vi "Main.vi"(11 "Module Admin":refnum<class "Delacor_lib_QMH_Cloneable Module Admin.lvclass">) -> ()   [LabVIEW 2020, in "DAQ AI.lvlib"]
doc: "This template is based off of the Queued Message Handler design pattern and the Queued Message Handler project template that ships with LabVIEW.\n\nThe main difference is that the queue is private to this module and communication between modules is performed via Broadcast and Request events.\n\nRequest events are wrapped in public API methods and are handled in the Event Handling Loop (EHL) of this VI. Any module can register for Broadcast events sent by this module. The EHL generates messages based on user interface actions.\n\nThe Message Handling Loop (MHL) processes messages generated by the EHL, or by other messages. The messages are string values, so new messages can be added easily to the Message Cases case structure in the MHL. Each message cluster can also provide an optional value for Message Data, which is a variant that can be converted to whatever message-specific data is required.\n_____\nBased on DQMH Dev Tools: Project Template 7.1.2.1547."
uses:
  DAQ AI.lvlib
  <vilib>/Delacor/Delacor QMH/Libraries/Cloneable Module Admin_class/Delacor_lib_QMH_Cloneable Module Admin.lvclass
  <vilib>/Delacor/Delacor QMH/Libraries/Message Queue_class/Delacor_lib_QMH_Message Queue.lvclass
  Module Data--cluster.ctl
  <vilib>/Utility/miscctls.llb/LVPointTypeDef.ctl
  <vilib>/Delacor/Delacor QMH/Libraries/Message Queue_class/Delacor_lib_QMH_Enqueue Message (Single).vi
  Stop Argument--cluster.ctl
  Get DAQ Analog Channel Argument--cluster.ctl
  <vilib>/DAQmx/read.llb/DAQmx Read (Analog DBL 1Chan 1Samp).vi
  Stop Acquisition Argument--cluster.ctl
  <vilib>/DAQmx/create/channels.llb/DAQmx Create Channel (AI-Voltage-Basic).vi
panel:
  out "task out":refnum<k21>
  out "DAQmx Physical Channel":tag
  out "error out":errorcluster
  out "Status":string
  in  "Simulate EHL Error":bool
  in  "Simulate MHL Error":bool
  # "Other processes communicate with this Module via its Public API (wrappers for its Request Events).\n\nThis Module communicates with other processes via its Broadcast Events.\nAny process that wants to receive these messages can register for this module's Broadcast events."
  # "This template is for the DQMH framework. See the block diagram for more information on how to use this template."
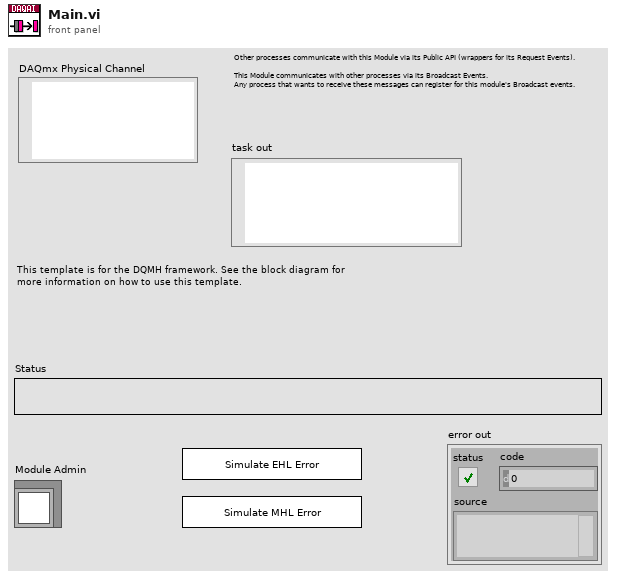
[diagram p1: front panel]
types:
  T1 = typedef "DAQ AI.lvlib/Request Events--cluster.ctl" = cluster{"Stop Module":refnum<user-event>, "Show Panel":refnum<user-event>, "Hide Panel":refnum<user-event>, "Show Diagram":refnum<user-event>, "Get Module Execution Status":refnum<user-event>, "Get DAQ Analog Channel":refnum<user-event>, "Get Acquisition Period":refnum<user-event>, "Stop Acquisition":refnum<user-event>}
  T2 = typedef "DAQ AI.lvlib/Module Data--cluster.ctl" = cluster{"Status":string, "DAQ Task":refnum<k21>}
  T3 = enum32{"invalid lock state", "Not Locked", "Locked (No Password)", "Password-protected"}
  T4 = typedef "DAQ AI.lvlib/Stop Argument--cluster.ctl" = cluster{"Module ID":i32, "Origin":string, "Exit via Stop Module Req?":bool, "Wait for Module to stop?":bool}
  T5 = typedef "DAQ AI.lvlib/Get DAQ Analog Channel Argument--cluster.ctl" = cluster{"Module ID":i32, "DAQmx Physical Channel":tag}
  T6 = typedef "DAQ AI.lvlib/Stop Acquisition Argument--cluster.ctl" = cluster{"Module ID":i32, "Dummy":bool}
  T7 = typedef "LVPointTypeDef.ctl" = cluster{"Horizontal":i16, "Vertical":i16}
  T8 = enum32{"Invalid", "Standard", "Closed", "Hidden", "Minimized", "Maximized"}
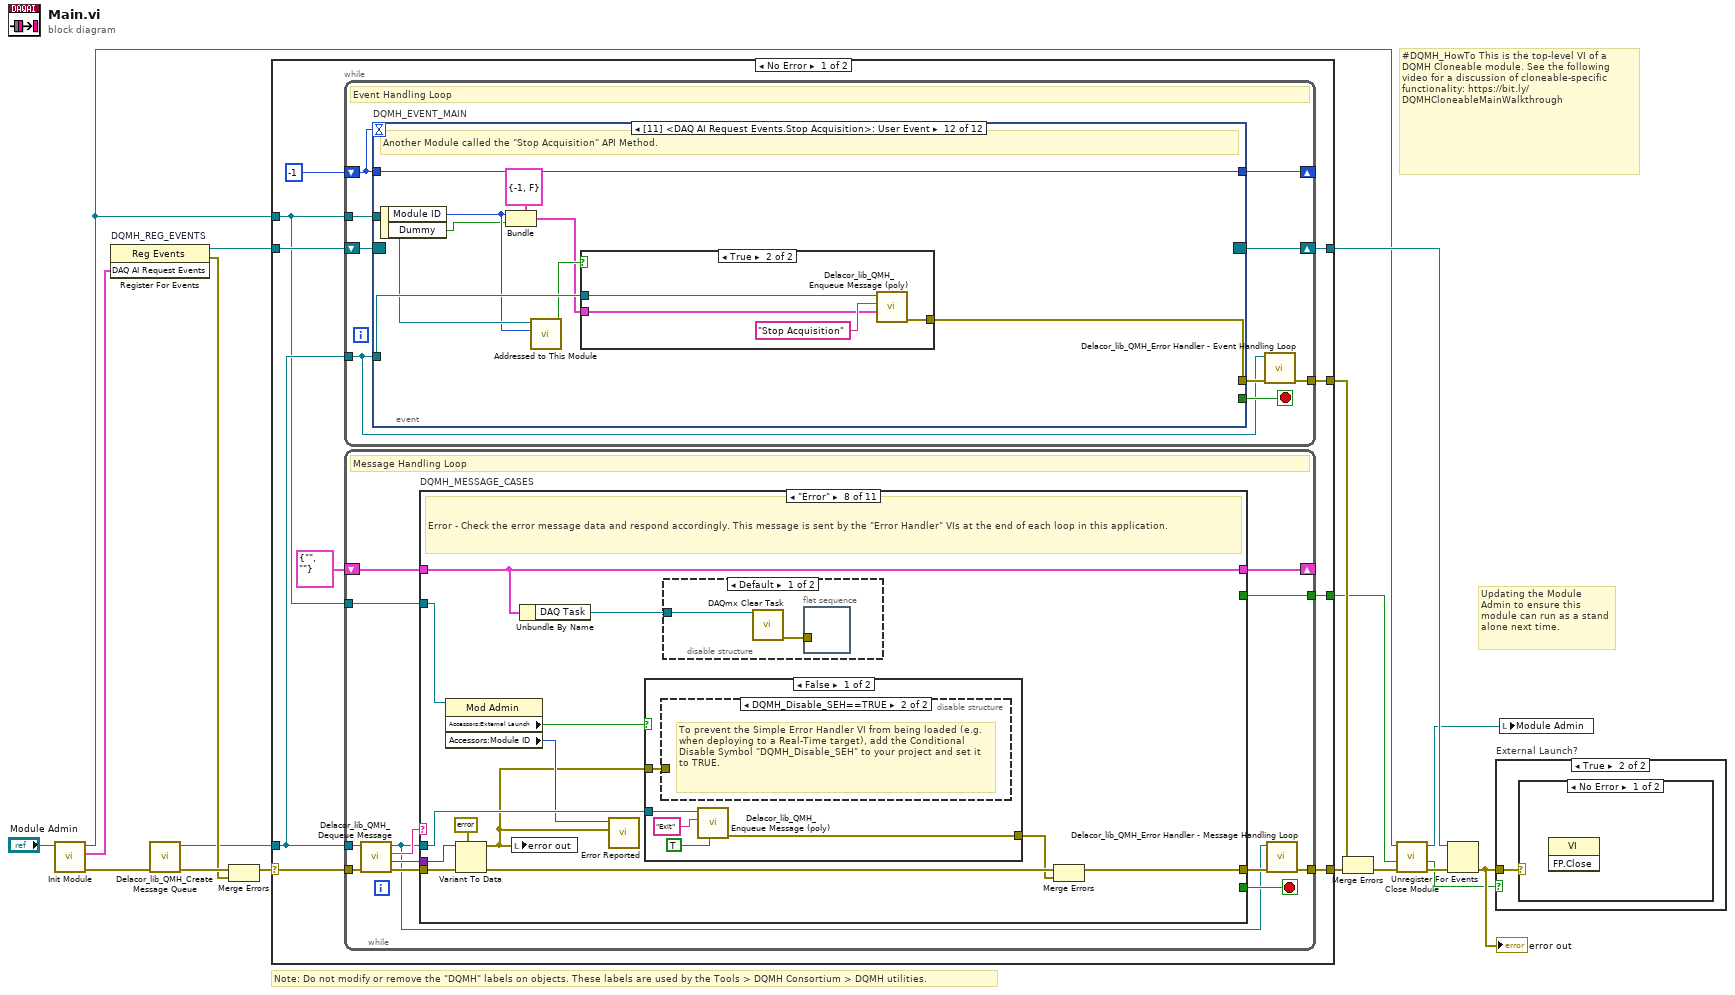
[diagram p0: block diagram]
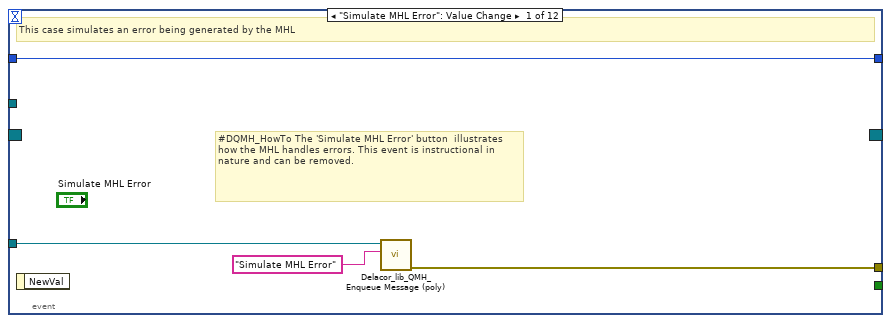
[diagram p2: hidden frame]
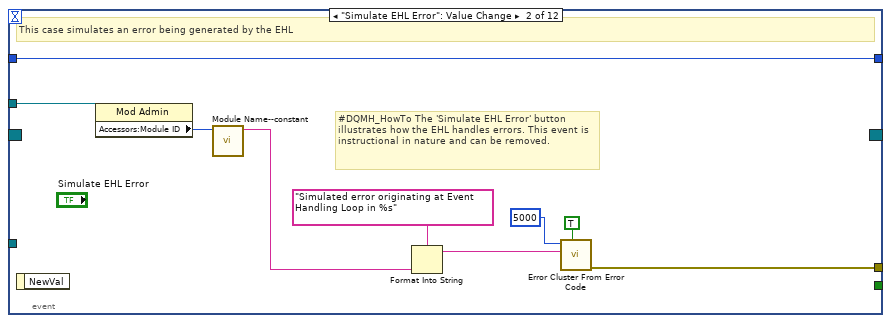
[diagram p3: hidden frame]
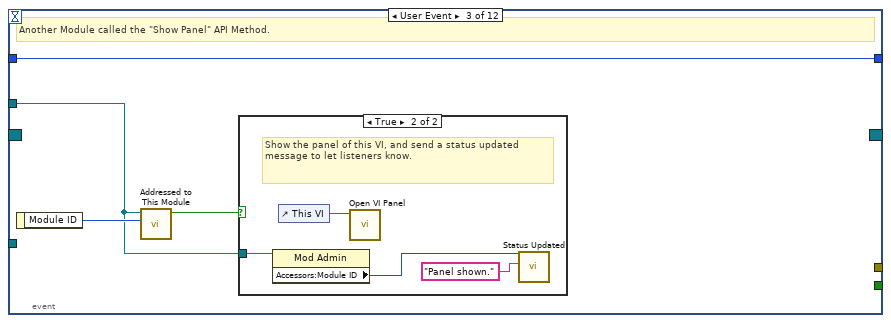
[diagram p4: hidden frame]
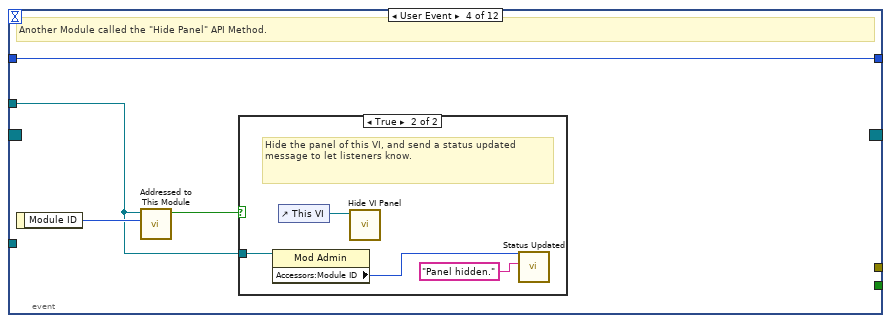
[diagram p6: hidden frame]
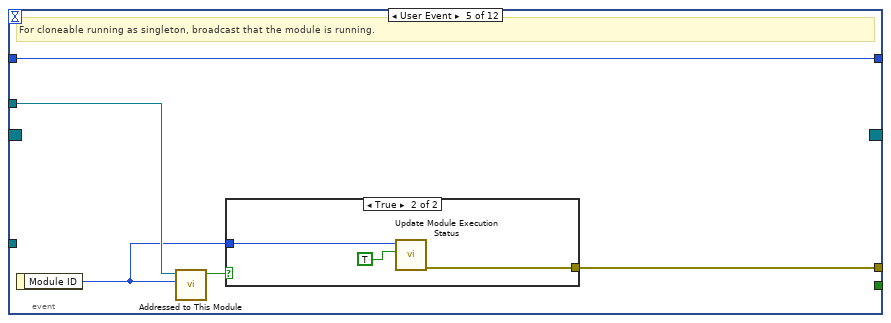
[diagram p8: hidden frame]
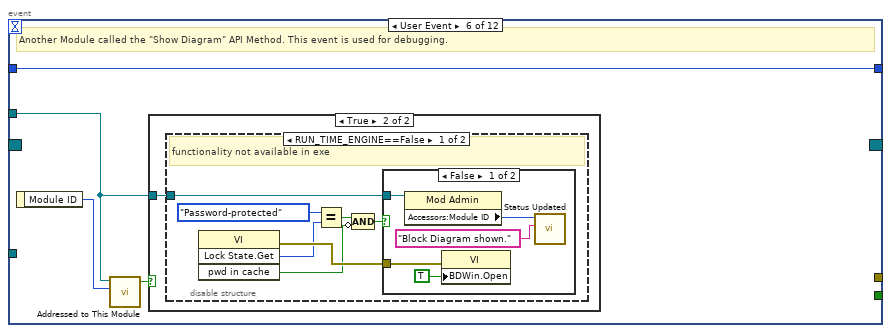
[diagram p10: hidden frame]
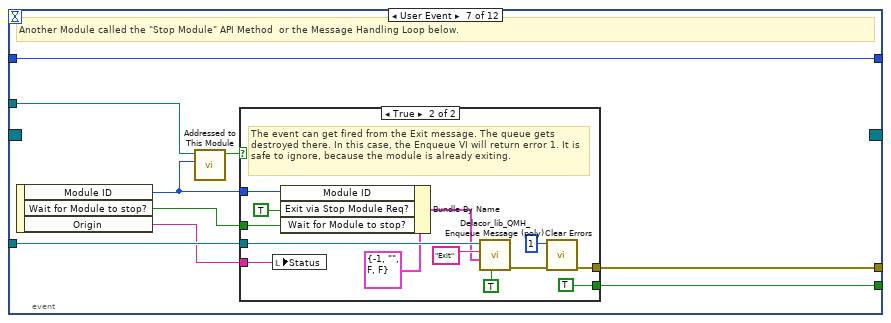
[diagram p14: hidden frame]
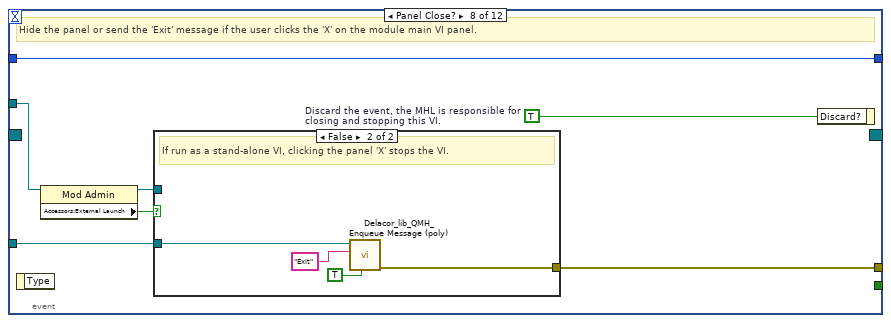
[diagram p16: hidden frame]
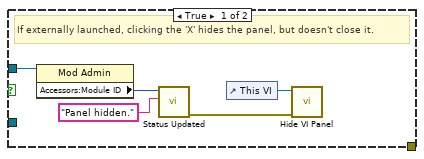
[diagram p17: hidden frame]
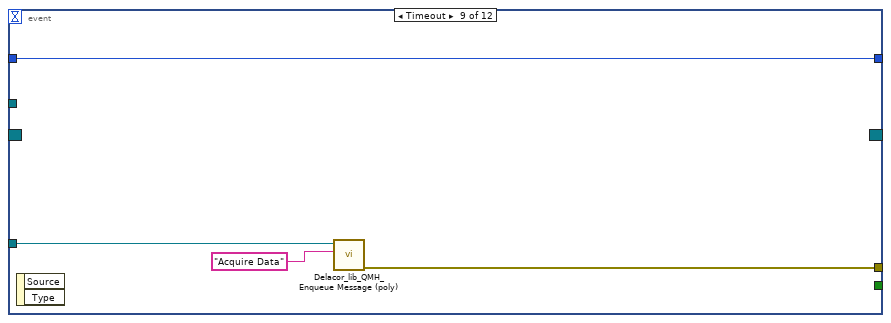
[diagram p18: hidden frame]
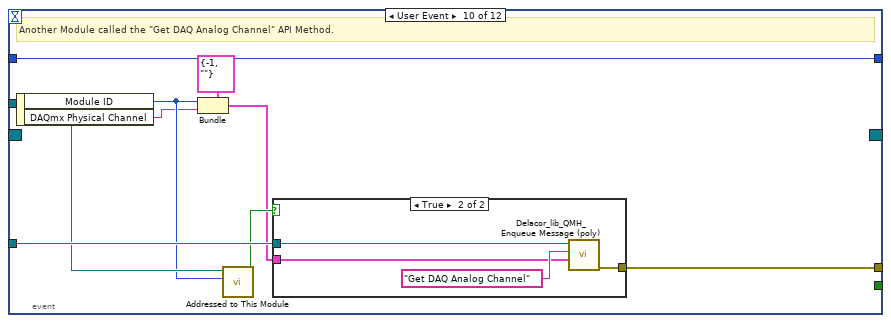
[diagram p19: hidden frame]
diagram:
  # "#DQMH_HowTo This is the top-level VI of a DQMH Cloneable module. See the following video for a discussion of cloneable-specific functionality: https://bit.ly/DQMHCloneableMainWalkthrough"
  # "Note: Do not modify or remove the \"DQMH\" labels on objects. These labels are used by the Tools > DQMH Consortium > DQMH utilities."
  # "Updating the Module Admin to ensure this module can run as a stand alone next time."
  n1 = call "Init Module.vi"("Cloneable Module Admin in"="Module Admin") -> ("error out"=w15:errorcluster, "DAQ AI Request Events"=w7:T1, "Cloneable Module Admin out"=w4:refnum<class "Delacor_lib_QMH_Cloneable Module Admin.lvclass">)  [unwired: 8 in]
  n2 = register-events "DQMH_REG_EVENTS"(w7) -> (reference out=w8:refnum<event-registration>, error out=w10:errorcluster)  [unwired: 2 in]
  n3 = call <vilib>:"Delacor_lib_QMH_Create Message Queue.vi"("error in"=w15) -> ("error out"=w12:errorcluster, "Message Queue"=w6:refnum<class "Delacor_lib_QMH_Message Queue.lvclass">)  [unwired: 9 in]
  n4 = Merge Errors(w12, w10) -> (w11:errorcluster)
  n5 = case shown="No Error" w11 {
    selector: w11 -> [w26 w322]
    tunnel: [w28 w321] -> w16
    tunnel: [w25 w320] -> w9
    tunnel: w8 -> [w23 w320]
    tunnel: w6 -> [w22 w313]
    tunnel: [w27 _] -> w17
    tunnel: w4 -> [w21 w316]
    tunnel: [w20 _] -> w2
    frame No Error {
      n6 = while {
        tunnel: w22 -> [w31]
        shift-right: [w34] -> w25
        shift-left: w23 -> [w35]
        tunnel: [w36] -> w27
        tunnel: w21 -> [w32]
        shift-right: [w30] -> _
        shift-left: -1 -> [w29]
        stop <- w33 stop-if-true
        # "Event Handling Loop"
        n7 = event "DQMH_EVENT_MAIN" shown="[11] <DAQ AI Request Events.Stop Acquisition>: User Event" {
          selector: w35 -> [_ _ _ _ _ _ _ _ _ _ _ _]
          dyn-events: [_ _ _ _ _ _ _ _ _ _ _ _] -> w34
          timeout: w29 -> [_ _ _ _ _ _ _ _ _ _ _ _]
          tunnel: [_ _ _ _ _ _ w96 _ _ _ _ _] -> w33
          tunnel: w31 -> [w40 _ _ _ _ _ w99 w117 w131 w141 _ w160]
          tunnel: [w41 w50 _ _ w71 _ w100 w120 w130 w134 _ w153] -> w37
          tunnel: w32 -> [_ w49 w52 w60 w69 w76 w98 w118 _ w139 w152 w158]
          tunnel: [w38 w42 w51 w59 w67 w75 w92 w114 w133 w142 w147 w161] -> w30
          tunnel: w29 -> [w38 w42 w51 w59 w67 w75 w92 w114 w133 w142 w148 w161]
          event "Simulate MHL Error": Value Change {
            # "#DQMH_HowTo The 'Simulate MHL Error' button  illustrates how the MHL handles errors. This event is instructional in nature and can be removed."
            # "This case simulates an error being generated by the MHL"
            n8 = event-data() -> ()  [unwired: 1 in, 1 out]
            n9 = call-poly <vilib>:"Delacor_lib_QMH_Enqueue Message (poly).vi"("Message"="Simulate MHL Error", "Message Queue in"=w40) -> ("error out"=w41:errorcluster)  [unwired: 8 in, 1 out]
          }
          event "Simulate EHL Error": Value Change {
            # "#DQMH_HowTo The 'Simulate EHL Error' button  illustrates how the EHL handles errors. This event is instructional in nature and can be removed."
            # "This case simulates an error being generated by the EHL"
            n10 = event-data() -> ()  [unwired: 1 in, 1 out]
            n11 = property on="Property Node" class="Mod Admin"(reference=w49) -> ("Accessors:Module ID"=w48:i32)  [unwired: 1 in, 2 out]
            n12 = call "Module Name--constant.vi"("Module ID"=w48) -> ("Module Name"=w43:string)  [unwired: 10 in]
            n13 = Format Into String(format string="Simulated error originating at Event Handling Loop in %s", w43) -> (resulting string=w46:string)  [unwired: 2 in, 1 out]
            n14 = call <vilib>:"Error Cluster From Error Code.vi"("show call chain? (False)"=TRUE, "error message (\"\")"=w46, "error code (0)"=5000) -> ("error out"=w50:errorcluster)  [unwired: 6 in]
          }
          event User Event {
            # "Another Module called the \"Show Panel\" API Method."
            n15 = event-data() -> ("Module ID"=w53:i32)  [unwired: 1 in]
            n16 = call "Addressed to This Module.vi"("Module ID from Argument"=w53, "Module Admin"=w52) -> ("Addressed to this instance?"=w54:bool)  [unwired: 8 in, 1 out]
            n17 = case shown="True" w54 {
              tunnel: w52 -> [_ w56]
              frame False {
              }
              frame True {
                # "Show the panel of this VI, and send a status updated message to let listeners know."
                n18 = property on="Property Node" class="Mod Admin"(reference=w56) -> ("Accessors:Module ID"=w55:i32)  [unwired: 1 in, 2 out]
                n19 = control-ref of="This VI"() -> (w58:refnum<vi>)
                n20 = call "Open VI Panel.vi"("VI"=w58) -> ()  [unwired: 10 in, 1 out]
                n21 = call "Status Updated.vi"("Status"="Panel shown." ("format string"), "Module ID"=w55) -> ()  [unwired: 9 in, 1 out]
              }
            }
          }
          event User Event {
            # "Another Module called the \"Hide Panel\" API Method."
            n22 = event-data() -> ("Module ID"=w61:i32)  [unwired: 1 in]
            n23 = call "Addressed to This Module.vi"("Module ID from Argument"=w61, "Module Admin"=w60) -> ("Addressed to this instance?"=w62:bool)  [unwired: 8 in, 1 out]
            n24 = case shown="True" w62 {
              tunnel: w60 -> [_ w64]
              frame False {
              }
              frame True {
                # "Hide the panel of this VI, and send a status updated message to let listeners know."
                n25 = property on="Property Node" class="Mod Admin"(reference=w64) -> ("Accessors:Module ID"=w63:i32)  [unwired: 1 in, 2 out]
                n26 = control-ref of="This VI"() -> (w66:refnum<vi>)
                n27 = call "Hide VI Panel.vi"("VI"=w66) -> ()  [unwired: 10 in, 1 out]
                n28 = call "Status Updated.vi"("Status"="Panel hidden." ("format string"), "Module ID"=w63) -> ()  [unwired: 9 in, 1 out]
              }
            }
          }
          event User Event {
            # "For cloneable running as singleton, broadcast that the module is running."
            n29 = event-data() -> ("Module ID"=w68:i32)  [unwired: 1 in]
            n30 = call "Addressed to This Module.vi"("Module ID from Argument"=w68, "Module Admin"=w69) -> ("Addressed to this instance?"=w70:bool)  [unwired: 8 in, 1 out]
            n31 = case shown="True" w70 {
              tunnel: [_ w74] -> w71
              tunnel: w68 -> [_ w73]
              frame False {
              }
              frame True {
                n32 = call "Update Module Execution Status.vi"("Running?"=TRUE, "Module ID"=w73) -> ("error out"=w74:errorcluster)  [unwired: 9 in]
              }
            }
          }
          event User Event {
            # "Another Module called the \"Show Diagram\" API Method. This event is used for debugging."
            n33 = event-data() -> ("Module ID"=w77:i32)  [unwired: 1 in]
            n34 = call "Addressed to This Module.vi"("Module ID from Argument"=w77, "Module Admin"=w76) -> ("Addressed to this instance?"=w78:bool)  [unwired: 8 in, 1 out]
            n35 = case shown="True" w78 {
              tunnel: w76 -> [_ w79]
              frame False {
              }
              frame True {
                n36 = disable-structure shown="RUN_TIME_ENGINE==False" {
                  disable-tunnel: w79 -> [w80 _]
                  frame condition #0 (active) {
                    # "functionality not available in exe"
                    n37 = invoke on="Invoke Node" class="VI" method="Lock State.Get"() -> (error out=w86:errorcluster, "Get Lock State"=w85:T3, "pwd in cache"=w82:bool)  [unwired: 4 in, 1 out]
                    n38 = Equal?(x=T3."Password-protected", y=w85) -> (x = y?=w83:bool)
                    n39 = Compound Arithmetic op=AND(w83, invert w82) -> (w81:bool)
                    n40 = case shown="False" w81 {
                      tunnel: w86 -> [w91 _]
                      tunnel: w80 -> [w88 _]
                      frame False {
                        n41 = property on="Property Node" class="Mod Admin"(reference=w88) -> ("Accessors:Module ID"=w87:i32)  [unwired: 1 in, 2 out]
                        n42 = property on="Property Node" class="VI"(error in=w91, "BDWin.Open"=TRUE ("Block Diagram Window:Open")) -> ()  [unwired: 1 in, 2 out]
                        n43 = call "Status Updated.vi"("Status"="Block Diagram shown." ("format string"), "Module ID"=w87) -> ()  [unwired: 9 in, 1 out]
                      }
                      frame True {
                        # "Password-protected VI, and the password is not in the cache. Do not show the diagram."
                      }
                    }
                  }
                  frame condition #1 {
                  }
                }
              }
            }
          }
          event User Event {
            # "Another Module called the \"Stop Module\" API Method  or the Message Handling Loop below."
            n44 = event-data() -> ("Module ID"=w94:i32, "Wait for Module to stop?"=w95:bool, "Origin"=w93:string)  [unwired: 1 in]
            n45 = call "Addressed to This Module.vi"("Module ID from Argument"=w94, "Module Admin"=w98) -> ("Addressed to this instance?"=w97:bool)  [unwired: 8 in, 1 out]
            n46 = case shown="True" w97 {
              tunnel: [_ w112] -> w100
              tunnel: w99 -> [_ w108]
              tunnel: [_ TRUE] -> w96
              tunnel: w95 -> [_ w103]
              tunnel: w94 -> [_ w105]
              tunnel: w93 -> [_ w101]
              frame False {
              }
              frame True {
                # "The event can get fired from the Exit message. The queue gets destroyed there. In this case, the Enqueue VI will return error 1. It is safe to ignore, because the module is already exiting."
                n47 = local write "Status"(w101) -> ()
                n48 = Bundle By Name(cluster=T4 {"Module ID"=-1, "Origin"="", "Exit via Stop Module Req?"=FALSE, "Wait for Module to stop?"=FALSE} ("Stop Argument"), "Module ID"=w105, "Exit via Stop Module Req?"=TRUE, "Wait for Module to stop?"=w103) -> (w102:T4)
                n49 = call-poly <vilib>:"Delacor_lib_QMH_Enqueue Message (poly).vi"("Priority Message? (F)"=TRUE, "Message Data"=w102, "Message"="Exit", "Message Queue in"=w108) -> ("error out"=w113:errorcluster)  [unwired: 6 in, 1 out]
                n50 = call <vilib>:"Clear Errors.vi"("error in (no error)"=w113, "specific error code to clear (0: all)"=1) -> ("error out"=w112:errorcluster)  [unwired: 4 in, 1 out]
              }
            }
          }
          event Panel Close? {
            w119 = TRUE  # Discard the event, the MHL is responsible for closing and stopping this VI.
            # "Hide the panel or send the 'Exit' message if the user clicks the 'X' on the module main VI panel."
            n51 = event-data() -> ()  [unwired: 1 in, 1 out]
            n52 = property on="Property Node" class="Mod Admin"(reference=w118) -> (reference out=w115:refnum<class "Delacor_lib_QMH_Cloneable Module Admin.lvclass">, "Accessors:External Launch"=w116:bool)  [unwired: 1 in, 1 out]
            n53 = case shown="False" w116 {
              tunnel: w117 -> [_ w128]
              tunnel: [_ w129] -> w120
              tunnel: w115 -> [w123 _]
              frame True {
                # "If externally launched, clicking the 'X' hides the panel, but doesn't close it."
                n54 = property on="Property Node" class="Mod Admin"(reference=w123) -> ("Accessors:Module ID"=w122:i32)  [unwired: 1 in, 2 out]
                n55 = call "Status Updated.vi"("Status"="Panel hidden." ("format string"), "Module ID"=w122) -> ("error out"=w121:errorcluster)  [unwired: 9 in]
                n56 = control-ref of="This VI"() -> (w125:refnum<vi>)
                n57 = call "Hide VI Panel.vi"("error in"=w121, "VI"=w125) -> ()  [unwired: 9 in, 1 out]
              }
              frame False {
                # "If run as a stand-alone VI, clicking the panel 'X' stops the VI."
                n58 = call-poly <vilib>:"Delacor_lib_QMH_Enqueue Message (poly).vi"("Priority Message? (F)"=TRUE, "Message"="Exit", "Message Queue in"=w128) -> ("error out"=w129:errorcluster)  [unwired: 7 in, 1 out]
              }
            }
            n59 = event-data ("Event Filter Node")("Discard?"=w119) -> ()  [unwired: 1 in, 1 out]
          }
          event Timeout {
            n60 = event-data() -> ()  [unwired: 1 in, 2 out]
            n61 = call-poly <vilib>:"Delacor_lib_QMH_Enqueue Message (poly).vi"("Message"="Acquire Data", "Message Queue in"=w131) -> ("error out"=w130:errorcluster)  [unwired: 8 in, 1 out]
          }
          event User Event {
            # "Another Module called the \"Get DAQ Analog Channel\" API Method."
            n62 = event-data() -> ("Module ID"=w136:i32, "DAQmx Physical Channel"=w135:tag)  [unwired: 1 in]
            n63 = Bundle(cluster=T5 {"Module ID"=-1, "DAQmx Physical Channel"=""} ("Get DAQ Analog Channel Argument"), "Module ID"=w136, "DAQmx Physical Channel"=w135) -> (w137:T5)
            n64 = call "Addressed to This Module.vi"("Module ID from Argument"=w136, "Module Admin"=w139) -> ("Addressed to this instance?"=w140:bool)  [unwired: 8 in, 1 out]
            n65 = case shown="True" w140 {
              tunnel: w141 -> [_ w146]
              tunnel: w137 -> [_ w144]
              tunnel: [_ w143] -> w134
              frame False {
              }
              frame True {
                n66 = call-poly <vilib>:"Delacor_lib_QMH_Enqueue Message (poly).vi"("Message Data"=w144, "Message"="Get DAQ Analog Channel", "Message Queue in"=w146) -> ("error out"=w143:errorcluster)  [unwired: 7 in, 1 out]
              }
            }
          }
          event User Event {
            # "Another Module called the \"Get Acquisition Period\" API Method."
            n67 = event-data() -> ("Module ID"=w151:i32, "Period [ms]"=w149:i32)  [unwired: 1 in]
            n68 = call "Addressed to This Module.vi"("Module ID from Argument"=w151, "Module Admin"=w152) -> ("Addressed to this instance?"=w150:bool)  [unwired: 8 in, 1 out]
            n69 = Select(t=w149, s=w150, f=w148) -> (s? t:f=w147:i32)
          }
          event User Event {
            # "Another Module called the \"Stop Acquisition\" API Method."
            n70 = event-data() -> ("Module ID"=w155:i32, "Dummy"=w154:bool)  [unwired: 1 in]
            n71 = Bundle(cluster=T6 {"Module ID"=-1, "Dummy"=FALSE} ("Stop Acquisition Argument"), "Module ID"=w155, "Dummy"=w154) -> (w156:T6)
            n72 = call "Addressed to This Module.vi"("Module ID from Argument"=w155, "Module Admin"=w158) -> ("Addressed to this instance?"=w159:bool)  [unwired: 8 in, 1 out]
            n73 = case shown="True" w159 {
              tunnel: w160 -> [_ w165]
              tunnel: w156 -> [_ w163]
              tunnel: [_ w162] -> w153
              frame False {
              }
              frame True {
                n74 = call-poly <vilib>:"Delacor_lib_QMH_Enqueue Message (poly).vi"("Message Data"=w163, "Message"="Stop Acquisition", "Message Queue in"=w165) -> ("error out"=w162:errorcluster)  [unwired: 7 in, 1 out]
              }
            }
          }
        }
        n75 = call-dynamic "Delacor_lib_QMH_Error Handler - Event Handling Loop.vi"("error in"=w37, "Message Queue in"=w31) -> ("dup error in"=w36:errorcluster)  [unwired: 8 in, 1 out]
      }
      n76 = while {
        tunnel: w22 -> [w166]
        shift-right: [w173] -> _
        shift-left: T2 {"Status"="", "DAQ Task"=""} ("Data Cluster") -> [w174]
        tunnel: w26 -> [w177]
        tunnel: [w175] -> w28
        tunnel: w21 -> [w168]
        tunnel: [w167] -> w20
        stop <- w172 stop-if-true
        # "Message Handling Loop"
        n77 = call-dynamic "Delacor_lib_QMH_Dequeue Message.vi"("error in"=w177, "Message Queue in"=w166) -> ("error out"=w176:errorcluster, "Message Data"=w170:variant, "Message"=w171:string, "Message Queue out"=w169:refnum<class "Delacor_lib_QMH_Message Queue.lvclass">)  [unwired: 6 in]
        n78 = case "DQMH_MESSAGE_CASES" shown="\"Error\"" w171 {
          selector: w171 -> [_ _ _ _ _ _ _ _ _ _ w302]
          tunnel: w169 -> [_ _ _ _ _ _ _ w253 _ w292 _]
          tunnel: w176 -> [w194 w198 w208 w222 w231 w237 w248 w261 w280 w298 w311]
          tunnel: [w192 w198 w202 w219 w230 w240 w248 w257 w279 w293 w312] -> w178
          tunnel: w174 -> [w188 w197 w204 w224 w229 w239 w247 w250 w277 w282 w309]
          tunnel: [w187 w197 w203 w224 w229 w239 w247 w250 w277 w282 w309] -> w173
          tunnel: [_ _ _ _ _ _ _ _ _ w291 _] -> w172
          tunnel: w170 -> [_ _ w207 _ _ _ _ w256 _ w289 _]
          tunnel: w168 -> [w184 _ _ w221 _ w233 _ w255 w275 w284 w308]
          tunnel: [_ _ _ _ _ _ _ _ _ w287 _] -> w167
          frame "Initialize" {
            w181 = "Initial Message" ("Initial Message")
            # "#DQMH_CodeNeeded - Initialize the appearance of the front panel."
            # "#DQMH_CodeNeeded - Initialize your state data here."
            # "Initialize - Any operation that needs to be done before the module can receive messages. Synchronize Caller Events.vi will inform Start Module.vi that the module has launched and is ready to receive messages. Module Did Init.vi will broadcast that the module initialized."
            n79 = call "Synchronize Caller Events.vi"("error in"=w194, "Module Admin"=w184) -> ("error out"=w193:errorcluster, "Module Admin out"=w183:refnum<class "Delacor_lib_QMH_Cloneable Module Admin.lvclass">)  [unwired: 8 in]
            n80 = property on="Property Node" class="Mod Admin" props=["Accessors:Module ID", "Accessors:External Launch"](reference=w183) -> ("Accessors:Module ID"=w180:i32)  [unwired: 1 in, 3 out]
            n81 = call "Module Name--constant.vi"("Module ID"=w180) -> ("Module Name"=w189:string)  [unwired: 10 in]
            n82 = property on="Property Node" class="VI"("Front Panel.Title"=w189) -> (reference out=w191:refnum<vi>, error out=w196:errorcluster)  [unwired: 2 in]
            n83 = invoke on="Invoke Node" class="VI" method="FP.Open"(reference=w191, error in=w196, "State"=T8."Hidden") -> (reference out=w190:refnum<vi>, error out=w195:errorcluster)  [unwired: 2 in, 3 out]
            n84 = Bundle By Name(cluster=w188, "Status"=w181) -> (w187:T2)
            n85 = invoke on="Invoke Node" class="VI" method="FP.Center"(reference=w190, error in=w195) -> ()  [unwired: 1 in, 3 out]
            n86 = property on="Pane" class="Pane"("Origin"=T7 {"Horizontal"=0, "Vertical"=0}) -> ()  [unwired: 2 in, 2 out]
            n87 = call "Module Name--constant.vi"("Module ID"=w180) -> ("Module Name"=w185:string)  [unwired: 10 in]
            n88 = call "Module Did Init.vi"("error in"=w193, "Initialized?"=TRUE, "Origin"=w185, "Module ID"=w180) -> ("error out"=w192:errorcluster)  [unwired: 7 in]
            "Status" <- w181
          }
          frame "---Module Specific---" {
            # "Separator -- The following cases handle messages specific to this Module."
          }
          frame "Get DAQ Analog Channel" {
            # "呼び出し元からアナログチャンネルを受け取ります。"
            n89 = Variant To Data(error in=w208, type=T5 {"Module ID"=-1, "DAQmx Physical Channel"=""} ("Get DAQ Analog Channel Argument"), Variant=w207) -> (data=w205:T5, error out=w201:errorcluster)
            n90 = Unbundle By Name(w205) -> ("DAQmx Physical Channel"=w200:tag)
            "DAQmx Physical Channel" <- w200
            n91 = disable-structure shown="Default" {
              disable-tunnel: [w214 w217] -> w202
              disable-tunnel: w201 -> [w211 w217]
              disable-tunnel: w200 -> [w210 _]
              disable-tunnel: [w209 _] -> w199
              frame condition #0 (active) {
                n92 = call <vilib>:"DAQmx Create Task.vi"("error in"=w211) -> ("task out"=w213:refnum<k21>, "error out"=w212:errorcluster)  [unwired: 13 in]
                n93 = call-poly <vilib>:"DAQmx Create Virtual Channel.vi"("task in"=w213, "physical channels"=w210, "error in"=w212) -> ("task out"=w216:refnum<k21>, "error out"=w215:errorcluster)  [unwired: 11 in]
                n94 = call <vilib>:"DAQmx Start Task.vi"("task/channels in"=w216, "error in"=w215) -> ("task out"=w209:refnum<k21>, "error out"=w214:errorcluster)  [unwired: 12 in]
              }
              frame condition #1 {
              }
            }
            "task out" <- w199
            n95 = Bundle By Name(cluster=w204, "DAQ Task"=w199) -> (w203:T2)
          }
          frame "Stop Acquisition" {
            # "データ集録を停止します。"
            n96 = Unbundle By Name(w224) -> ("DAQ Task"=w223:refnum<k21>)
            n97 = disable-structure shown="Default" {
              disable-tunnel: w223 -> [w226 _]
              disable-tunnel: w222 -> [w225 _]
              frame condition #0 (active) {
                n98 = call <vilib>:"DAQmx Stop Task.vi"("task/channels in"=w226, "error in"=w225) -> ("task out"=w228:refnum<k21>, "error out"=w227:errorcluster)  [unwired: 12 in]
                n99 = call <vilib>:"DAQmx Clear Task.vi"("task in"=w228, "error in"=w227) -> ()  [unwired: 13 in, 1 out]
              }
              frame condition #1 {
              }
            }
            n100 = property class="Mod Admin"(reference=w221) -> ("Accessors:Module ID"=w220:i32)  [unwired: 1 in, 2 out]
            n101 = call "Clear DAQ Task.vi"("Dummy"=TRUE, "Module ID"=w220) -> ("error out"=w219:errorcluster)  [unwired: 9 in]
          }
          frame "---Copy This Frame---" {
            # "Duplicate this frame when creating new messages.  Change this comment in the duplicated frame to describe this message."
            n102 = Merge Errors(w231) -> (w230:errorcluster)
          }
          frame "Acquire Data" {
            # "イベントストラクチャがタイムアウトしたらデータを集録します。"
            n103 = Unbundle By Name(w239) -> ("DAQ Task"=w238:refnum<k21>)
            n104 = property class="Mod Admin"(reference=w233) -> ("Accessors:Module ID"=w232:i32)  [unwired: 1 in, 2 out]
            n105 = disable-structure shown="DAQ_AI_SImulation==TRUE" {
              disable-tunnel: w238 -> [w244 _]
              disable-tunnel: w237 -> [w243 w246]
              disable-tunnel: [w242 w245] -> w236
              disable-tunnel: [w241 w246] -> w235
              frame condition #0 (active) {
                n106 = call-poly <vilib>:"DAQmx Read.vi"("task/channels in"=w244, "error in"=w243) -> ("data"=w242:dbl, "error out"=w241:errorcluster)  [unwired: 11 in, 1 out]
              }
              frame condition #1 {
                n107 = Random Number (0-1)() -> (number: 0 to 1=w245:dbl)
              }
            }
            n108 = call "Send Acquired Data.vi"("error in"=w235, "Value"=w236, "Module ID"=w232) -> ("error out"=w234:errorcluster)  [unwired: 8 in]
            n109 = Merge Errors(w234) -> (w240:errorcluster)
          }
          frame "---Exit and Error Handling---" {
            # "Separator - the following cases handle errors and exit messages."
          }
          frame "Error" {
            # "Error - Check the error message data and respond accordingly. This message is sent by the \"Error Handler\" VIs at the end of each loop in this application."
            n110 = property on="Property Node" class="Mod Admin"(reference=w255) -> ("Accessors:External Launch"=w254:bool, "Accessors:Module ID"=w252:i32)  [unwired: 1 in, 2 out]
            n111 = Variant To Data(error in=w261, type=errorcluster {"status"=FALSE, "code"=0, "source"=""} ("error constant"), Variant=w256) -> (data=w251:errorcluster, error out=w259:errorcluster)
            n112 = local write "error out"(w251) -> ()
            n113 = Unbundle By Name(w250) -> ("DAQ Task"=w249:refnum<k21>)
            n114 = call "Error Reported.vi"("Error"=w251, "Module ID"=w252) -> ()  [unwired: 9 in, 1 out]
            n115 = case shown="False" w254 {
              tunnel: [w268 _] -> w258
              tunnel: w253 -> [w266 _]
              tunnel: w251 -> [w267 _]
              frame False {
                n116 = disable-structure shown="DQMH_Disable_SEH==TRUE" {
                  disable-tunnel: w267 -> [w269 _]
                  frame condition #0 {
                    # "If the module is running standalone, then pop up an error dialog and call the \"Exit\" message."
                    n117 = call <vilib>:"Simple Error Handler.vi"("error in (no error)"=w269) -> ()  [unwired: 4 in, 5 out]
                  }
                  frame condition #1 (active) {
                    # "To prevent the Simple Error Handler VI from being loaded (e.g. when deploying to a Real-Time target), add the Conditional Disable Symbol \"DQMH_Disable_SEH\" to your project and set it to TRUE."
                  }
                }
                n118 = call-poly <vilib>:"Delacor_lib_QMH_Enqueue Message (poly).vi"("Priority Message? (F)"=TRUE, "Message"="Exit", "Message Queue in"=w266) -> ("error out"=w268:errorcluster)  [unwired: 7 in, 1 out]
              }
              frame True {
                # "If the module was launched externally, calling the Error Reported broadcast VI is the only action performed by the \"Error\" message. The module's caller can then process the error appropriately."
              }
            }
            n119 = disable-structure shown="Default" {
              disable-tunnel: w249 -> [w263 _]
              frame condition #0 (active) {
                n120 = call <vilib>:"DAQmx Clear Task.vi"("task in"=w263) -> ("error out"=w262:errorcluster)  [unwired: 14 in]
                n121 = flat-sequence {
                  tunnel: w262 -> [_]
                  frame #0 {
                  }
                }
              }
              frame condition #1 {
              }
            }
            n122 = Merge Errors(w259, w258) -> (w257:errorcluster)
          }
          frame "Simulate MHL Error" {
            # "#DQMH_HowTo The 'Simulate MHL Error' button  illustrates how the MHL handles errors. This event is instructional in nature and can be removed."
            # "Simulate an error occurring at the MHL"
            n123 = property on="Property Node" class="Mod Admin"(reference=w275) -> ("Accessors:Module ID"=w276:i32)  [unwired: 1 in, 2 out]
            n124 = call "Module Name--constant.vi"("Module ID"=w276) -> ("Module Name"=w271:string)  [unwired: 10 in]
            n125 = Format Into String(format string="Simulated error originating at Message Handling Loop in %s", w271) -> (resulting string=w272:string)  [unwired: 2 in, 1 out]
            n126 = call <vilib>:"Error Cluster From Error Code.vi"("show call chain? (False)"=TRUE, "error message (\"\")"=w272, "error code (0)"=5001) -> ("error out"=w278:errorcluster)  [unwired: 6 in]
            n127 = Merge Errors(w280, w278) -> (w279:errorcluster)
          }
          frame "Exit" {
            w290 = 91  # 91: not all Exit messages will have an argument
            w291 = TRUE  # Stop the VI
            # "Release the message queue reference"
            # "#DQMH_CodeNeeded - Add any required cleanup code here."
            # "Exit - Exit the application."
            n128 = Variant To Data(error in=w298, type=T4 {"Module ID"=-1, "Origin"="", "Exit via Stop Module Req?"=FALSE, "Wait for Module to stop?"=FALSE} ("Stop Argument"), Variant=w289) -> (data=w286:T4, error out=w294:errorcluster)
            n129 = call <vilib>:"Clear Errors.vi"("error in (no error)"=w294, "specific error code to clear (0: all)"=w290) -> ("error out"=w297:errorcluster)  [unwired: 4 in, 1 out]
            n130 = property on="Property Node" class="Mod Admin"(reference=w284) -> ("Accessors:Module ID"=w283:i32)  [unwired: 1 in, 2 out]
            n131 = control-ref of="This VI"() -> (w285:refnum<vi>)
            n132 = call-dynamic "Delacor_lib_QMH_Release Message Queue.vi"("error in"=w297, "Message Queue"=w292) -> ("error out"=w296:errorcluster)  [unwired: 9 in]
            n133 = call "Handle Exit.vi"("Stop Argument"=w286, "Module Admin in"=w284, "VI reference"=w285) -> ("error out"=w295:errorcluster, "Wait for Stop?"=w287:bool)  [unwired: 7 in]
            n134 = Merge Errors(w296, w295) -> (w293:errorcluster)
            n135 = Unbundle By Name(w282) -> ("DAQ Task"=w281:refnum<k21>)
            n136 = call "Error Reported.vi"("Error"=w293, "Module ID"=w283) -> ()  [unwired: 9 in, 1 out]
            n137 = disable-structure shown="Default" {
              disable-tunnel: w281 -> [w300 _]
              frame condition #0 (active) {
                n138 = call <vilib>:"DAQmx Clear Task.vi"("task in"=w300) -> ("error out"=w299:errorcluster)  [unwired: 14 in]
                n139 = flat-sequence {
                  tunnel: w299 -> [_]
                  frame #0 {
                  }
                }
              }
              frame condition #1 {
              }
            }
          }
          frame Default {
            # "'Default' case only runs if there is a message that isn't defined in any of the other cases.  Output a programming error."
            n140 = property on="Property Node" class="Mod Admin"(reference=w308) -> ("Accessors:Module ID"=w307:i32)  [unwired: 1 in, 2 out]
            n141 = call "Module Name--constant.vi"("Module ID"=w307) -> ("Module Name"=w301:string)  [unwired: 10 in]
            n142 = Format Into String(format string="The invalid message string \"%s\" was received in the Message Handling Loop for module \"%s\".", w302, w301) -> (resulting string=w304:string)  [unwired: 2 in, 1 out]
            n143 = call <vilib>:"Error Cluster From Error Code.vi"("show call chain? (False)"=TRUE, "error message (\"\")"=w304, "error code (0)"=1) -> ("error out"=w310:errorcluster)  [unwired: 6 in]
            n144 = Merge Errors(w311, w310) -> (w312:errorcluster)
          }
        }
        n145 = call-dynamic "Delacor_lib_QMH_Error Handler - Message Handling Loop.vi"("error in"=w178, "Message Queue in"=w169) -> ("dup error in"=w175:errorcluster)  [unwired: 8 in, 1 out]
      }
    }
    frame Error {
      n146 = call "Synchronize Caller Events.vi"("Module Admin"=w316) -> ("Module Admin out"=w315:refnum<class "Delacor_lib_QMH_Cloneable Module Admin.lvclass">)  [unwired: 9 in, 1 out]
      n147 = property on="Property Node" class="Mod Admin"(reference=w315) -> ("Accessors:Module ID"=w314:i32)  [unwired: 1 in, 2 out]
      n148 = call-dynamic "Delacor_lib_QMH_Release Message Queue.vi"("error in"=w322, "Message Queue"=w313) -> ("error out"=w321:errorcluster)  [unwired: 9 in]
      n149 = call "Module Name--constant.vi"("Module ID"=w314) -> ("Module Name"=w319:string)  [unwired: 10 in]
      n150 = Format Into String(format string="An error occurred during initialization. %s is no longer running.", w319) -> (resulting string=w317:string)  [unwired: 2 in, 1 out]
      n151 = call "Error Reported.vi"("Additional Information"=w317, "Error"=w321, "Module ID"=w314) -> ()  [unwired: 8 in, 1 out]
    }
  }
  n152 = Merge Errors(w17, w16) -> (w18:errorcluster)
  n153 = call "Close Module.vi"("error in"=w18, "Wait for stop?"=w2, "Module Admin in"=w4) -> ("error out"=w14:errorcluster, "External Launch"=w1:bool, "Module Admin out"=w3:refnum<class "Delacor_lib_QMH_Cloneable Module Admin.lvclass">)  [unwired: 6 in]
  n154 = Unregister For Events(event registration refnum=w9, error in=w14) -> (error out=w13:errorcluster)
  "error out" <- w13
  n155 = case "External Launch?" shown="True" w1 {
    tunnel: w13 -> [_ w323]
    frame False {
    }
    frame True {
      n156 = case shown="No Error" w323 {
        frame No Error {
          n157 = invoke class="VI" method="FP.Close"() -> ()  [unwired: 3 in, 3 out]
        }
        frame Error {
          n158 = disable-structure shown="Default" {
            frame condition #0 (active) {
              n159 = invoke class="VI" method="FP.Open"("Activate"=TRUE ("Activate?")) -> ()  [unwired: 4 in, 5 out]
            }
            frame condition #1 {
              # "Don't show panel on error if running inside a built EXE."
            }
          }
        }
      }
    }
  }
  n160 = local write "Module Admin"(w3) -> ()
